vi "FindProjectPath.vi"(8 "error in (no error)":errorcluster, 11 "Library/Class Name":string) -> (0 "error out":errorcluster, 2 "Found?":bool, 3 "Project Path":path)   [LabVIEW 2019]
uses:
  <vilib>/SLL Toolkit/SLL String/SLL String.lvlib
  Hawkeye.lvlib
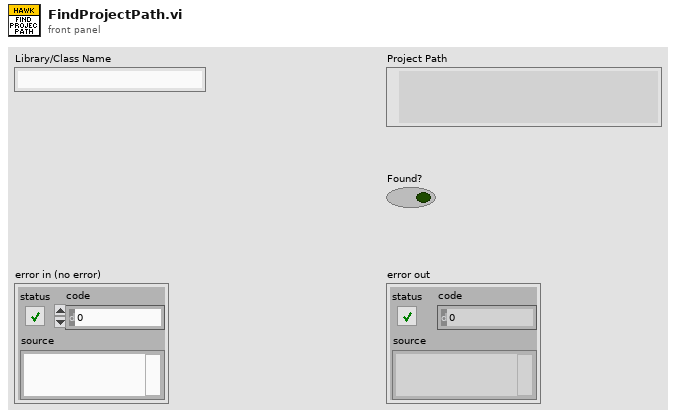
[diagram p1: front panel]
types:
  T1 = typedef "Hawkeye.lvlib/HawkeyePathConfigs.ctl" = cluster{"GlobalIncludePaths":path[], "GlobalExcludePaths":path[], "BuildSpecsIncludePaths":path[], "ActualDepsIncludePaths":path[], "WorkspacePath":path, "SourceFolderPaths":path[], "ChangedFilesLogpaths":map{string, path}}
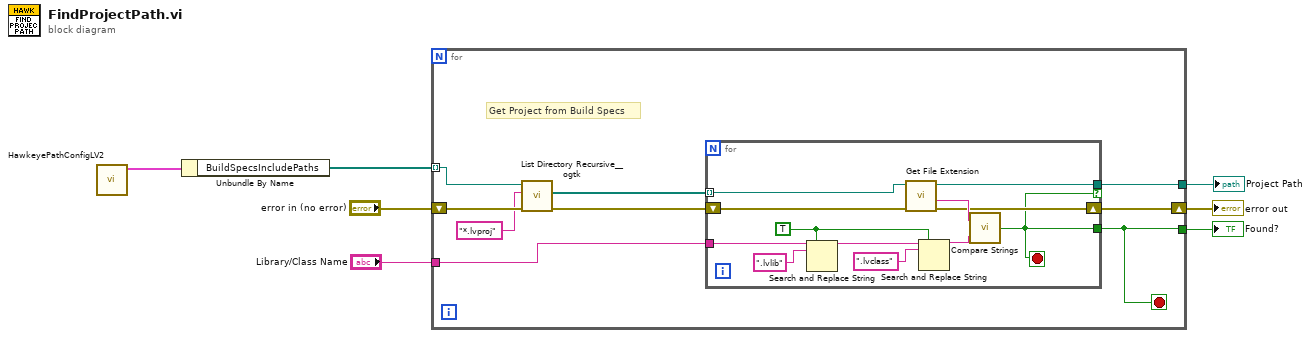
[diagram p0: block diagram]
diagram:
  n1 = call "HawkeyePathConfigLV2.vi"() -> ("Hawkeye Path Config Out"=w2:T1)  [unwired: 11 in]
  n2 = Unbundle By Name(w2) -> ("BuildSpecsIncludePaths"=w1:path[])
  n3 = for {
    tunnel: [w15] -> w6
    tunnel: [w8] -> w5
    tunnel: "Library/Class Name" -> [w13]
    shift-right: [w10] -> w3
    shift-left: "error in (no error)" -> [w16]
    tunnel: w1 -> [w9] mode=indexing
    stop <- w8 stop-if-true
    # "Get Project from Build Specs"
    n4 = call <userlib>:"List Directory Recursive__ogtk.vi"("error in (no error)"=w16, "pattern"="*.lvproj", "Path"=w9) -> ("error out"=w14:errorcluster, "file paths"=w12:path[])  [unwired: 5 in, 2 out]
    n5 = for {
      tunnel: w12 -> [w27] mode=indexing
      tunnel: w13 -> [w18]
      shift-right: [w23] -> w10
      shift-left: w14 -> [w28]
      tunnel: [w22] -> w15 if=w21
      tunnel: [w21] -> w8
      stop <- w21 stop-if-true
      w17 = TRUE ("replace all? (F)")
      n6 = Search and Replace String(replace all?=w17, input string=w18, search string=".lvlib") -> (result string=w19:string)  [unwired: 5 in, 3 out]
      n7 = call <vilib>:"Get File Extension.vi"("error in (no error)"=w28, "file"=w27) -> ("error out"=w23:errorcluster, "filename without extension"=w25:string, "dup file"=w22:path)  [unwired: 5 in, 2 out]
      n8 = Search and Replace String(replace all?=w17, input string=w19, search string=".lvclass") -> (result string=w24:string)  [unwired: 5 in, 3 out]
      n9 = call <vilib>:"Compare Strings.vi"("y"=w24, "x"=w25) -> ("Equal?"=w21:bool)
    }
  }
  "Project Path" <- w6
  "Found?" <- w5
  "error out" <- w3
